vi "Close VI Reference.vi"(8 "error in":errorcluster, 11 "VI Reference":refnum<vi>) -> (0 "error out":errorcluster)   [LabVIEW 2020]
doc: "Closing the VI reference is important. Otherwise, error 1357 can occur in certain situations.\n\nError message of error code 1357:\n\"LabVIEW: (Hex 0x54D) A LabVIEW file from that path already exists in memory, or exists within a project library already in memory.\""
panel:
  # "Development\ncontrols/indicators useful for development and testing, but which are not outputs of the VI"
  # "Input\nInputs to the VI"
  # "Output\nOutputs of the VI"
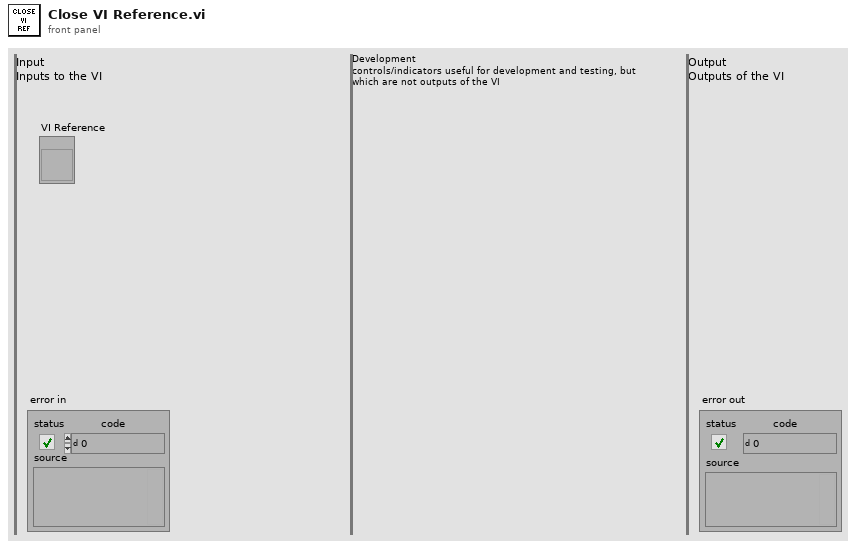
[diagram p1: front panel]
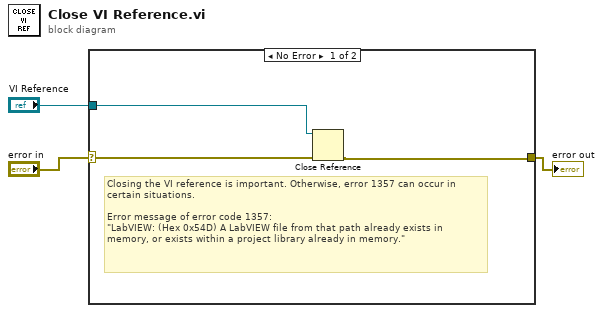
[diagram p0: block diagram]
diagram:
  n1 = case shown="No Error" "error in" {
    selector: "error in" -> [w6 w7]
    tunnel: [w5 w7] -> w2
    tunnel: "VI Reference" -> [w4 _]
    frame No Error {
      # "Closing the VI reference is important. Otherwise, error 1357 can occur in certain situations.\n\nError message of error code 1357:\n\"LabVIEW: (Hex 0x54D) A LabVIEW file from that path already exists in memory, or exists within a project library already in memory.\""
      n2 = Close Reference(reference=w4, error in (no error)=w6) -> (error out=w5:errorcluster)
    }
    frame Error {
    }
  }
  "error out" <- w2
